vi "Generate Report work with Zee 2.vi"(6 "Graph Properties":T2(array[cluster])=[{"Plot Traces"=[{"Color Box"=4652800, "Boolean"=TRUE, "List 2"=39, "Boolean 2"=TRUE, "Boolean 3"=FALSE, "Offset"=0.0, "Gain"=1.0}, {"Color Box"=16733696, "Boolean"=TRUE, "List 2"=33, "Boolean 2"=FALSE, "Boolean 3"=FALSE, "Offset"=0.0, "Gain"=1.0}, {"Color Box"=393436, "Boolean"=TRUE, "List 2"=36, "Boolean 2"=FALSE, "Boolean 3"=FALSE, "Offset"=0.0, "Gain"=1.0}], "Gain Calculations"={"Threshold Trace"=39, "Min Thresh/%"=0.2, "Max Thresh/%"=0.8, "Gain calculated by dividing"=33, "Gain Range"=enum."Best Est", "Pre-peak-ms"=30.0, "by"=39}, "Impulse Plane"=enum."LARP", "Impulse Direction"=TRUE}, {"Plot Traces"=[{"Color Box"=4652800, "Boolean"=TRUE, "List 2"=39, "Boolean 2"=FALSE, "Boolean 3"=FALSE, "Offset"=0.0, "Gain"=1.0}, {"Color Box"=16733696, "Boolean"=TRUE, "List 2"=33, "Boolean 2"=TRUE, "Boolean 3"=FALSE, "Offset"=0.0, "Gain"=1.0}, {"Color Box"=393436, "Boolean"=TRUE, "List 2"=36, "Boolean 2"=TRUE, "Boolean 3"=FALSE, "Offset"=0.0, "Gain"=1.0}], "Gain Calculations"={"Threshold Trace"=39, "Min Thresh/%"=0.2, "Max Thresh/%"=0.8, "Gain calculated by dividing"=33, "Gain Range"=enum."Best Est", "Pre-peak-ms"=30.0, "by"=39}, "Impulse Plane"=enum."LARP", "Impulse Direction"=FALSE}, {"Plot Traces"=[{"Color Box"=4652800, "Boolean"=TRUE, "List 2"=42, "Boolean 2"=TRUE, "Boolean 3"=FALSE, "Offset"=0.0, "Gain"=1.0}, {"Color Box"=16733696, "Boolean"=TRUE, "List 2"=33, "Boolean 2"=FALSE, "Boolean 3"=FALSE, "Offset"=0.0, "Gain"=1.0}, {"Color Box"=393436, "Boolean"=TRUE, "List 2"=36, "Boolean 2"=FALSE, "Boolean 3"=FALSE, "Offset"=0.0, "Gain"=1.0}], "Gain Calculations"={"Threshold Trace"=42, "Min Thresh/%"=0.2, "Max Thresh/%"=0.8, "Gain calculated by dividing"=36, "Gain Range"=enum."Best Est", "Pre-peak-ms"=30.0, "by"=42}, "Impulse Plane"=enum."LARP", "Impulse Direction"=TRUE}, {"Plot Traces"=[{"Color Box"=4652800, "Boolean"=TRUE, "List 2"=42, "Boolean 2"=FALSE, "Boolean 3"=FALSE, "Offset"=0.0, "Gain"=1.0}, {"Color Box"=16733696, "Boolean"=TRUE, "List 2"=33, "Boolean 2"=TRUE, "Boolean 3"=FALSE, "Offset"=0.0, "Gain"=1.0}, {"Color Box"=393436, "Boolean"=TRUE, "List 2"=36, "Boolean 2"=TRUE, "Boolean 3"=FALSE, "Offset"=0.0, "Gain"=1.0}], "Gain Calculations"={"Threshold Trace"=42, "Min Thresh/%"=0.2, "Max Thresh/%"=0.8, "Gain calculated by dividing"=36, "Gain Range"=enum."Best Est", "Pre-peak-ms"=30.0, "by"=42}, "Impulse Plane"=enum."LARP", "Impulse Direction"=FALSE}, {"Plot Traces"=[{"Color Box"=4652800, "Boolean"=TRUE, "List 2"=38, "Boolean 2"=TRUE, "Boolean 3"=FALSE, "Offset"=0.0, "Gain"=1.0}, {"Color Box"=16733696, "Boolean"=TRUE, "List 2"=32, "Boolean 2"=FALSE, "Boolean 3"=FALSE, "Offset"=0.0, "Gain"=1.0}, {"Color Box"=393436, "Boolean"=TRUE, "List 2"=35, "Boolean 2"=FALSE, "Boolean 3"=FALSE, "Offset"=0.0, "Gain"=1.0}], "Gain Calculations"={"Threshold Trace"=38, "Min Thresh/%"=0.2, "Max Thresh/%"=0.8, "Gain calculated by dividing"=32, "Gain Range"=enum."Best Est", "Pre-peak-ms"=30.0, "by"=38}, "Impulse Plane"=enum."LARP", "Impulse Direction"=FALSE}, {"Plot Traces"=[{"Color Box"=4652800, "Boolean"=TRUE, "List 2"=38, "Boolean 2"=FALSE, "Boolean 3"=FALSE, "Offset"=0.0, "Gain"=1.0}, {"Color Box"=16733696, "Boolean"=TRUE, "List 2"=32, "Boolean 2"=TRUE, "Boolean 3"=FALSE, "Offset"=0.0, "Gain"=1.0}, {"Color Box"=393436, "Boolean"=TRUE, "List 2"=35, "Boolean 2"=TRUE, "Boolean 3"=FALSE, "Offset"=0.0, "Gain"=1.0}], "Gain Calculations"={"Threshold Trace"=38, "Min Thresh/%"=0.2, "Max Thresh/%"=0.8, "Gain calculated by dividing"=32, "Gain Range"=enum."Best Est", "Pre-peak-ms"=30.0, "by"=38}, "Impulse Plane"=enum."LARP", "Impulse Direction"=TRUE}, {"Plot Traces"=[{"Color Box"=4652800, "Boolean"=TRUE, "List 2"=41, "Boolean 2"=TRUE, "Boolean 3"=FALSE, "Offset"=0.0, "Gain"=1.0}, {"Color Box"=16733696, "Boolean"=TRUE, "List 2"=32, "Boolean 2"=FALSE, "Boolean 3"=FALSE, "Offset"=0.0, "Gain"=1.0}, {"Color Box"=393436, "Boolean"=TRUE, "List 2"=35, "Boolean 2"=FALSE, "Boolean 3"=FALSE, "Offset"=0.0, "Gain"=1.0}], "Gain Calculations"={"Threshold Trace"=41, "Min Thresh/%"=0.2, "Max Thresh/%"=0.8, "Gain calculated by dividing"=35, "Gain Range"=enum."Best Est", "Pre-peak-ms"=30.0, "by"=41}, "Impulse Plane"=enum."LARP", "Impulse Direction"=FALSE}, {"Plot Traces"=[{"Color Box"=4652800, "Boolean"=TRUE, "List 2"=41, "Boolean 2"=FALSE, "Boolean 3"=FALSE, "Offset"=0.0, "Gain"=1.0}, {"Color Box"=16733696, "Boolean"=TRUE, "List 2"=32, "Boolean 2"=TRUE, "Boolean 3"=FALSE, "Offset"=0.0, "Gain"=1.0}, {"Color Box"=393436, "Boolean"=TRUE, "List 2"=35, "Boolean 2"=TRUE, "Boolean 3"=FALSE, "Offset"=0.0, "Gain"=1.0}], "Gain Calculations"={"Threshold Trace"=41, "Min Thresh/%"=0.2, "Max Thresh/%"=0.8, "Gain calculated by dividing"=35, "Gain Range"=enum."Best Est", "Pre-peak-ms"=30.0, "by"=41}, "Impulse Plane"=enum."LARP", "Impulse Direction"=TRUE}, {"Plot Traces"=[{"Color Box"=4652800, "Boolean"=TRUE, "List 2"=39, "Boolean 2"=FALSE, "Boolean 3"=FALSE, "Offset"=0.0, "Gain"=1.0}, {"Color Box"=16733696, "Boolean"=TRUE, "List 2"=33, "Boolean 2"=TRUE, "Boolean 3"=FALSE, "Offset"=0.0, "Gain"=1.0}, {"Color Box"=393436, "Boolean"=TRUE, "List 2"=36, "Boolean 2"=TRUE, "Boolean 3"=FALSE, "Offset"=0.0, "Gain"=1.0}], "Gain Calculations"={"Threshold Trace"=39, "Min Thresh/%"=0.2, "Max Thresh/%"=0.8, "Gain calculated by dividing"=33, "Gain Range"=enum."Best Est", "Pre-peak-ms"=30.0, "by"=39}, "Impulse Plane"=enum."RALP", "Impulse Direction"=TRUE}, {"Plot Traces"=[{"Color Box"=4652800, "Boolean"=TRUE, "List 2"=39, "Boolean 2"=TRUE, "Boolean 3"=FALSE, "Offset"=0.0, "Gain"=1.0}, {"Color Box"=16733696, "Boolean"=TRUE, "List 2"=33, "Boolean 2"=FALSE, "Boolean 3"=FALSE, "Offset"=0.0, "Gain"=1.0}, {"Color Box"=393436, "Boolean"=TRUE, "List 2"=36, "Boolean 2"=FALSE, "Boolean 3"=FALSE, "Offset"=0.0, "Gain"=1.0}], "Gain Calculations"={"Threshold Trace"=39, "Min Thresh/%"=0.2, "Max Thresh/%"=0.8, "Gain calculated by dividing"=33, "Gain Range"=enum."Best Est", "Pre-peak-ms"=30.0, "by"=39}, "Impulse Plane"=enum."RALP", "Impulse Direction"=FALSE}, {"Plot Traces"=[{"Color Box"=4652800, "Boolean"=TRUE, "List 2"=42, "Boolean 2"=FALSE, "Boolean 3"=FALSE, "Offset"=0.0, "Gain"=1.0}, {"Color Box"=16733696, "Boolean"=TRUE, "List 2"=33, "Boolean 2"=TRUE, "Boolean 3"=FALSE, "Offset"=0.0, "Gain"=1.0}, {"Color Box"=393436, "Boolean"=TRUE, "List 2"=36, "Boolean 2"=TRUE, "Boolean 3"=FALSE, "Offset"=0.0, "Gain"=1.0}], "Gain Calculations"={"Threshold Trace"=42, "Min Thresh/%"=0.2, "Max Thresh/%"=0.8, "Gain calculated by dividing"=36, "Gain Range"=enum."Best Est", "Pre-peak-ms"=30.0, "by"=42}, "Impulse Plane"=enum."RALP", "Impulse Direction"=TRUE}, {"Plot Traces"=[{"Color Box"=4652800, "Boolean"=TRUE, "List 2"=42, "Boolean 2"=TRUE, "Boolean 3"=FALSE, "Offset"=0.0, "Gain"=1.0}, {"Color Box"=16733696, "Boolean"=TRUE, "List 2"=33, "Boolean 2"=FALSE, "Boolean 3"=FALSE, "Offset"=0.0, "Gain"=1.0}, {"Color Box"=393436, "Boolean"=TRUE, "List 2"=36, "Boolean 2"=FALSE, "Boolean 3"=FALSE, "Offset"=0.0, "Gain"=1.0}], "Gain Calculations"={"Threshold Trace"=42, "Min Thresh/%"=0.2, "Max Thresh/%"=0.8, "Gain calculated by dividing"=36, "Gain Range"=enum."Best Est", "Pre-peak-ms"=30.0, "by"=42}, "Impulse Plane"=enum."RALP", "Impulse Direction"=FALSE}, {"Plot Traces"=[{"Color Box"=4652800, "Boolean"=TRUE, "List 2"=38, "Boolean 2"=FALSE, "Boolean 3"=FALSE, "Offset"=0.0, "Gain"=1.0}, {"Color Box"=16733696, "Boolean"=TRUE, "List 2"=32, "Boolean 2"=TRUE, "Boolean 3"=FALSE, "Offset"=0.0, "Gain"=1.0}, {"Color Box"=393436, "Boolean"=TRUE, "List 2"=35, "Boolean 2"=TRUE, "Boolean 3"=FALSE, "Offset"=0.0, "Gain"=1.0}], "Gain Calculations"={"Threshold Trace"=38, "Min Thresh/%"=0.2, "Max Thresh/%"=0.8, "Gain calculated by dividing"=32, "Gain Range"=enum."Best Est", "Pre-peak-ms"=30.0, "by"=38}, "Impulse Plane"=enum."RALP", "Impulse Direction"=TRUE}, {"Plot Traces"=[{"Color Box"=4652800, "Boolean"=TRUE, "List 2"=38, "Boolean 2"=TRUE, "Boolean 3"=FALSE, "Offset"=0.0, "Gain"=1.0}, {"Color Box"=16733696, "Boolean"=TRUE, "List 2"=32, "Boolean 2"=FALSE, "Boolean 3"=FALSE, "Offset"=0.0, "Gain"=1.0}, {"Color Box"=393436, "Boolean"=TRUE, "List 2"=35, "Boolean 2"=FALSE, "Boolean 3"=FALSE, "Offset"=0.0, "Gain"=1.0}], "Gain Calculations"={"Threshold Trace"=38, "Min Thresh/%"=0.2, "Max Thresh/%"=0.8, "Gain calculated by dividing"=32, "Gain Range"=enum."Best Est", "Pre-peak-ms"=30.0, "by"=38}, "Impulse Plane"=enum."RALP", "Impulse Direction"=FALSE}, {"Plot Traces"=[{"Color Box"=4652800, "Boolean"=TRUE, "List 2"=41, "Boolean 2"=FALSE, "Boolean 3"=FALSE, "Offset"=0.0, "Gain"=1.0}, {"Color Box"=16733696, "Boolean"=TRUE, "List 2"=32, "Boolean 2"=TRUE, "Boolean 3"=FALSE, "Offset"=0.0, "Gain"=1.0}, {"Color Box"=393436, "Boolean"=TRUE, "List 2"=35, "Boolean 2"=TRUE, "Boolean 3"=FALSE, "Offset"=0.0, "Gain"=1.0}], "Gain Calculations"={"Threshold Trace"=41, "Min Thresh/%"=0.2, "Max Thresh/%"=0.8, "Gain calculated by dividing"=35, "Gain Range"=enum."Best Est", "Pre-peak-ms"=30.0, "by"=41}, "Impulse Plane"=enum."RALP", "Impulse Direction"=TRUE}, {"Plot Traces"=[{"Color Box"=4652800, "Boolean"=TRUE, "List 2"=41, "Boolean 2"=TRUE, "Boolean 3"=FALSE, "Offset"=0.0, "Gain"=1.0}, {"Color Box"=16733696, "Boolean"=TRUE, "List 2"=32, "Boolean 2"=FALSE, "Boolean 3"=FALSE, "Offset"=0.0, "Gain"=1.0}, {"Color Box"=393436, "Boolean"=TRUE, "List 2"=35, "Boolean 2"=FALSE, "Boolean 3"=FALSE, "Offset"=0.0, "Gain"=1.0}], "Gain Calculations"={"Threshold Trace"=41, "Min Thresh/%"=0.2, "Max Thresh/%"=0.8, "Gain calculated by dividing"=35, "Gain Range"=enum."Best Est", "Pre-peak-ms"=30.0, "by"=41}, "Impulse Plane"=enum."RALP", "Impulse Direction"=FALSE}] {"Gain Calculations"."by" items=["Hx Position-in-Head", "Hy Position-in-Head", "Hz Position-in-Head", "Hx Velocity-in-Head", "Hy Velocity-in-Head", "Hz Velocity-in-Head", "Hl Velocity-in-Head", "Hr Velocity-in-Head", "Lx Position-in-Head", "Ly Position-in-Head", "Lz Position-in-Head", "Lx Velocity-in-Head", "Ly Velocity-in-Head", "Lz Velocity-in-Head", "Ll Velocity-in-Head", "Lr Velocity-in-Head", "Rx Position-in-Head", "Ry Position-in-Head", "Rz Position-in-Head", "Rx Velocity-in-Head", "Ry Velocity-in-Head", "Rz Velocity-in-Head", "Rl Velocity-in-Head", "Rr Velocity-in-Head", "Button", "Ascension X", "Ascension X Vel", "Ascension Y", "Ascension Y Vel", "Ascension Z", "Ascension Z Vel", " ", "Lx Velocity-in-Eye", "Ly Velocity-in-Eye", "Lz Velocity-in-Eye", "Rx Velocity-in-Eye", "Ry Velocity-in-Eye", "Rz Velocity-in-Eye", "Hx Velocity-in-Left Eye", "Hy Velocity-in-Left Eye", "Hz Velocity-in-Left Eye", "Hx Velocity-in-Right-Eye", "Hy Velocity-in-Right-Eye", "Hz Velocity-in-Right-Eye"]; "Gain Calculations"."Pre-peak-ms" format="%.2f"; "Gain Calculations"."Gain calculated by dividing" items=["Hx Position-in-Head", "Hy Position-in-Head", "Hz Position-in-Head", "Hx Velocity-in-Head", "Hy Velocity-in-Head", "Hz Velocity-in-Head", "Hl Velocity-in-Head", "Hr Velocity-in-Head", "Lx Position-in-Head", "Ly Position-in-Head", "Lz Position-in-Head", "Lx Velocity-in-Head", "Ly Velocity-in-Head", "Lz Velocity-in-Head", "Ll Velocity-in-Head", "Lr Velocity-in-Head", "Rx Position-in-Head", "Ry Position-in-Head", "Rz Position-in-Head", "Rx Velocity-in-Head", "Ry Velocity-in-Head", "Rz Velocity-in-Head", "Rl Velocity-in-Head", "Rr Velocity-in-Head", "Button", "Ascension X", "Ascension X Vel", "Ascension Y", "Ascension Y Vel", "Ascension Z", "Ascension Z Vel", " ", "Lx Velocity-in-Eye", "Ly Velocity-in-Eye", "Lz Velocity-in-Eye", "Rx Velocity-in-Eye", "Ry Velocity-in-Eye", "Rz Velocity-in-Eye", "Hx Velocity-in-Left Eye", "Hy Velocity-in-Left Eye", "Hz Velocity-in-Left Eye", "Hx Velocity-in-Right-Eye", "Hy Velocity-in-Right-Eye", "Hz Velocity-in-Right-Eye"]; "Gain Calculations"."Max Thresh/%" format="%.2f"; "Gain Calculations"."Min Thresh/%" format="%.2f"; "Gain Calculations"."Threshold Trace" items=["Hx Position-in-Head", "Hy Position-in-Head", "Hz Position-in-Head", "Hx Velocity-in-Head", "Hy Velocity-in-Head", "Hz Velocity-in-Head", "Hl Velocity-in-Head", "Hr Velocity-in-Head", "Lx Position-in-Head", "Ly Position-in-Head", "Lz Position-in-Head", "Lx Velocity-in-Head", "Ly Velocity-in-Head", "Lz Velocity-in-Head", "Ll Velocity-in-Head", "Lr Velocity-in-Head", "Rx Position-in-Head", "Ry Position-in-Head", "Rz Position-in-Head", "Rx Velocity-in-Head", "Ry Velocity-in-Head", "Rz Velocity-in-Head", "Rl Velocity-in-Head", "Rr Velocity-in-Head", "Button", "Ascension X", "Ascension X Vel", "Ascension Y", "Ascension Y Vel", "Ascension Z", "Ascension Z Vel", " ", "Lx Velocity-in-Eye", "Ly Velocity-in-Eye", "Lz Velocity-in-Eye", "Rx Velocity-in-Eye", "Ry Velocity-in-Eye", "Rz Velocity-in-Eye", "Hx Velocity-in-Left Eye", "Hy Velocity-in-Left Eye", "Hz Velocity-in-Left Eye", "Hx Velocity-in-Right-Eye", "Hy Velocity-in-Right-Eye", "Hz Velocity-in-Right-Eye"]; "Plot Traces"."Gain" format="%.1f"; "Plot Traces"."Offset" format="%.1f"; "Plot Traces"."List 2" items=["Hx Position-in-Head", "Hy Position-in-Head", "Hz Position-in-Head", "Hx Velocity-in-Head", "Hy Velocity-in-Head", "Hz Velocity-in-Head", "Hl Velocity-in-Head", "Hr Velocity-in-Head", "Lx Position-in-Head", "Ly Position-in-Head", "Lz Position-in-Head", "Lx Velocity-in-Head", "Ly Velocity-in-Head", "Lz Velocity-in-Head", "Ll Velocity-in-Head", "Lr Velocity-in-Head", "Rx Position-in-Head", "Ry Position-in-Head", "Rz Position-in-Head", "Rx Velocity-in-Head", "Ry Velocity-in-Head", "Rz Velocity-in-Head", "Rl Velocity-in-Head", "Rr Velocity-in-Head", "Button", "Ascension X", "Ascension X Vel", "Ascension Y", "Ascension Y Vel", "Ascension Z", "Ascension Z Vel", " ", "Lx Velocity-in-Eye", "Ly Velocity-in-Eye", "Lz Velocity-in-Eye", "Rx Velocity-in-Eye", "Ry Velocity-in-Eye", "Rz Velocity-in-Eye", "Hx Velocity-in-Left Eye", "Hy Velocity-in-Left Eye", "Hz Velocity-in-Left Eye", "Hx Velocity-in-Right-Eye", "Hy Velocity-in-Right-Eye", "Hz Velocity-in-Right-Eye"]}, 8 "Impulse Positions":T4(array[cluster])=[{"Start"=5147, "End"=5187, "Impulse Plane"=enum."Yaw", "Impulse Direction +ve?"=TRUE, "Time offset"=0, "Amplitude offset"=0.0}, {"Start"=5544, "End"=5586, "Impulse Plane"=enum."Yaw", "Impulse Direction +ve?"=FALSE, "Time offset"=0, "Amplitude offset"=0.0}, {"Start"=5784, "End"=5826, "Impulse Plane"=enum."Yaw", "Impulse Direction +ve?"=FALSE, "Time offset"=0, "Amplitude offset"=0.0}, {"Start"=6210, "End"=6250, "Impulse Plane"=enum."Yaw", "Impulse Direction +ve?"=TRUE, "Time offset"=0, "Amplitude offset"=0.0}, {"Start"=6409, "End"=6449, "Impulse Plane"=enum."Yaw", "Impulse Direction +ve?"=TRUE, "Time offset"=0, "Amplitude offset"=0.0}, {"Start"=6617, "End"=6657, "Impulse Plane"=enum."Yaw", "Impulse Direction +ve?"=TRUE, "Time offset"=0, "Amplitude offset"=0.0}, {"Start"=6856, "End"=6898, "Impulse Plane"=enum."Yaw", "Impulse Direction +ve?"=FALSE, "Time offset"=0, "Amplitude offset"=0.0}, {"Start"=7143, "End"=7185, "Impulse Plane"=enum."Yaw", "Impulse Direction +ve?"=FALSE, "Time offset"=0, "Amplitude offset"=0.0}, {"Start"=7918, "End"=7958, "Impulse Plane"=enum."Yaw", "Impulse Direction +ve?"=TRUE, "Time offset"=0, "Amplitude offset"=0.0}, {"Start"=8170, "End"=8210, "Impulse Plane"=enum."Yaw", "Impulse Direction +ve?"=TRUE, "Time offset"=0, "Amplitude offset"=0.0}, {"Start"=9145, "End"=9185, "Impulse Plane"=enum."Yaw", "Impulse Direction +ve?"=TRUE, "Time offset"=0, "Amplitude offset"=0.0}, {"Start"=9434, "End"=9476, "Impulse Plane"=enum."Yaw", "Impulse Direction +ve?"=FALSE, "Time offset"=0, "Amplitude offset"=0.0}, {"Start"=9732, "End"=9774, "Impulse Plane"=enum."Yaw", "Impulse Direction +ve?"=FALSE, "Time offset"=0, "Amplitude offset"=0.0}, {"Start"=10023, "End"=10065, "Impulse Plane"=enum."Yaw", "Impulse Direction +ve?"=FALSE, "Time offset"=0, "Amplitude offset"=0.0}, {"Start"=10545, "End"=10585, "Impulse Plane"=enum."Yaw", "Impulse Direction +ve?"=TRUE, "Time offset"=0, "Amplitude offset"=0.0}, {"Start"=11028, "End"=11068, "Impulse Plane"=enum."Yaw", "Impulse Direction +ve?"=TRUE, "Time offset"=0, "Amplitude offset"=0.0}, {"Start"=11326, "End"=11366, "Impulse Plane"=enum."Yaw", "Impulse Direction +ve?"=TRUE, "Time offset"=0, "Amplitude offset"=0.0}, {"Start"=11654, "End"=11696, "Impulse Plane"=enum."Yaw", "Impulse Direction +ve?"=FALSE, "Time offset"=0, "Amplitude offset"=0.0}, {"Start"=11983, "End"=12025, "Impulse Plane"=enum."Yaw", "Impulse Direction +ve?"=FALSE, "Time offset"=0, "Amplitude offset"=0.0}, {"Start"=12228, "End"=12270, "Impulse Plane"=enum."Yaw", "Impulse Direction +ve?"=FALSE, "Time offset"=0, "Amplitude offset"=0.0}, {"Start"=12796, "End"=12836, "Impulse Plane"=enum."Yaw", "Impulse Direction +ve?"=TRUE, "Time offset"=0, "Amplitude offset"=0.0}, {"Start"=13150, "End"=13190, "Impulse Plane"=enum."Yaw", "Impulse Direction +ve?"=TRUE, "Time offset"=0, "Amplitude offset"=0.0}, {"Start"=13420, "End"=13460, "Impulse Plane"=enum."Yaw", "Impulse Direction +ve?"=TRUE, "Time offset"=0, "Amplitude offset"=0.0}, {"Start"=14002, "End"=14044, "Impulse Plane"=enum."Yaw", "Impulse Direction +ve?"=FALSE, "Time offset"=0, "Amplitude offset"=0.0}, {"Start"=14311, "End"=14351, "Impulse Plane"=enum."Yaw", "Impulse Direction +ve?"=TRUE, "Time offset"=0, "Amplitude offset"=0.0}, {"Start"=14611, "End"=14651, "Impulse Plane"=enum."Yaw", "Impulse Direction +ve?"=TRUE, "Time offset"=0, "Amplitude offset"=0.0}, {"Start"=15419, "End"=15461, "Impulse Plane"=enum."Yaw", "Impulse Direction +ve?"=FALSE, "Time offset"=0, "Amplitude offset"=0.0}, {"Start"=15681, "End"=15723, "Impulse Plane"=enum."Yaw", "Impulse Direction +ve?"=FALSE, "Time offset"=0, "Amplitude offset"=0.0}, {"Start"=15969, "End"=16009, "Impulse Plane"=enum."Yaw", "Impulse Direction +ve?"=TRUE, "Time offset"=0, "Amplitude offset"=0.0}, {"Start"=16818, "End"=16858, "Impulse Plane"=enum."Yaw", "Impulse Direction +ve?"=TRUE, "Time offset"=0, "Amplitude offset"=0.0}, {"Start"=17055, "End"=17097, "Impulse Plane"=enum."Yaw", "Impulse Direction +ve?"=FALSE, "Time offset"=0, "Amplitude offset"=0.0}, {"Start"=18327, "End"=18369, "Impulse Plane"=enum."Yaw", "Impulse Direction +ve?"=FALSE, "Time offset"=0, "Amplitude offset"=0.0}, {"Start"=18817, "End"=18859, "Impulse Plane"=enum."Yaw", "Impulse Direction +ve?"=FALSE, "Time offset"=0, "Amplitude offset"=0.0}, {"Start"=19049, "End"=19089, "Impulse Plane"=enum."Yaw", "Impulse Direction +ve?"=TRUE, "Time offset"=0, "Amplitude offset"=0.0}, {"Start"=21122, "End"=21188, "Impulse Plane"=enum."LARP", "Impulse Direction +ve?"=TRUE, "Time offset"=0, "Amplitude offset"=0.0}, {"Start"=21362, "End"=21430, "Impulse Plane"=enum."LARP", "Impulse Direction +ve?"=TRUE, "Time offset"=0, "Amplitude offset"=0.0}, {"Start"=21593, "End"=21661, "Impulse Plane"=enum."LARP", "Impulse Direction +ve?"=TRUE, "Time offset"=0, "Amplitude offset"=0.0}, {"Start"=22327, "End"=22395, "Impulse Plane"=enum."LARP", "Impulse Direction +ve?"=TRUE, "Time offset"=0, "Amplitude offset"=0.0}, {"Start"=22537, "End"=22604, "Impulse Plane"=enum."LARP", "Impulse Direction +ve?"=TRUE, "Time offset"=0, "Amplitude offset"=0.0}, {"Start"=22777, "End"=22844, "Impulse Plane"=enum."LARP", "Impulse Direction +ve?"=TRUE, "Time offset"=0, "Amplitude offset"=0.0}, {"Start"=23019, "End"=23086, "Impulse Plane"=enum."LARP", "Impulse Direction +ve?"=TRUE, "Time offset"=0, "Amplitude offset"=0.0}, {"Start"=23291, "End"=23358, "Impulse Plane"=enum."LARP", "Impulse Direction +ve?"=TRUE, "Time offset"=0, "Amplitude offset"=0.0}, {"Start"=23566, "End"=23631, "Impulse Plane"=enum."LARP", "Impulse Direction +ve?"=TRUE, "Time offset"=0, "Amplitude offset"=0.0}, {"Start"=23861, "End"=23929, "Impulse Plane"=enum."LARP", "Impulse Direction +ve?"=FALSE, "Time offset"=0, "Amplitude offset"=0.0}, {"Start"=24575, "End"=24641, "Impulse Plane"=enum."LARP", "Impulse Direction +ve?"=TRUE, "Time offset"=0, "Amplitude offset"=0.0}, {"Start"=24924, "End"=24993, "Impulse Plane"=enum."LARP", "Impulse Direction +ve?"=TRUE, "Time offset"=0, "Amplitude offset"=0.0}, {"Start"=25253, "End"=25318, "Impulse Plane"=enum."LARP", "Impulse Direction +ve?"=TRUE, "Time offset"=0, "Amplitude offset"=0.0}, {"Start"=25536, "End"=25602, "Impulse Plane"=enum."LARP", "Impulse Direction +ve?"=TRUE, "Time offset"=0, "Amplitude offset"=0.0}, {"Start"=26288, "End"=26350, "Impulse Plane"=enum."LARP", "Impulse Direction +ve?"=FALSE, "Time offset"=0, "Amplitude offset"=0.0}, {"Start"=26578, "End"=26645, "Impulse Plane"=enum."LARP", "Impulse Direction +ve?"=FALSE, "Time offset"=0, "Amplitude offset"=0.0}, {"Start"=26940, "End"=27006, "Impulse Plane"=enum."LARP", "Impulse Direction +ve?"=FALSE, "Time offset"=0, "Amplitude offset"=0.0}, {"Start"=27202, "End"=27271, "Impulse Plane"=enum."LARP", "Impulse Direction +ve?"=FALSE, "Time offset"=0, "Amplitude offset"=0.0}, {"Start"=27477, "End"=27544, "Impulse Plane"=enum."LARP", "Impulse Direction +ve?"=TRUE, "Time offset"=0, "Amplitude offset"=0.0}, {"Start"=27709, "End"=27775, "Impulse Plane"=enum."LARP", "Impulse Direction +ve?"=TRUE, "Time offset"=0, "Amplitude offset"=0.0}, {"Start"=27926, "End"=27993, "Impulse Plane"=enum."LARP", "Impulse Direction +ve?"=TRUE, "Time offset"=0, "Amplitude offset"=0.0}, {"Start"=28185, "End"=28251, "Impulse Plane"=enum."LARP", "Impulse Direction +ve?"=TRUE, "Time offset"=0, "Amplitude offset"=0.0}, {"Start"=28672, "End"=28736, "Impulse Plane"=enum."LARP", "Impulse Direction +ve?"=FALSE, "Time offset"=0, "Amplitude offset"=0.0}, {"Start"=29607, "End"=29677, "Impulse Plane"=enum."LARP", "Impulse Direction +ve?"=TRUE, "Time offset"=0, "Amplitude offset"=0.0}, {"Start"=29829, "End"=29898, "Impulse Plane"=enum."LARP", "Impulse Direction +ve?"=TRUE, "Time offset"=0, "Amplitude offset"=0.0}, {"Start"=30266, "End"=30335, "Impulse Plane"=enum."LARP", "Impulse Direction +ve?"=TRUE, "Time offset"=0, "Amplitude offset"=0.0}, {"Start"=30991, "End"=31057, "Impulse Plane"=enum."LARP", "Impulse Direction +ve?"=FALSE, "Time offset"=0, "Amplitude offset"=0.0}, {"Start"=32437, "End"=32505, "Impulse Plane"=enum."LARP", "Impulse Direction +ve?"=TRUE, "Time offset"=0, "Amplitude offset"=0.0}, {"Start"=33030, "End"=33097, "Impulse Plane"=enum."LARP", "Impulse Direction +ve?"=FALSE, "Time offset"=0, "Amplitude offset"=0.0}, {"Start"=33660, "End"=33727, "Impulse Plane"=enum."LARP", "Impulse Direction +ve?"=FALSE, "Time offset"=0, "Amplitude offset"=0.0}, {"Start"=34390, "End"=34456, "Impulse Plane"=enum."LARP", "Impulse Direction +ve?"=FALSE, "Time offset"=0, "Amplitude offset"=0.0}, {"Start"=34672, "End"=34738, "Impulse Plane"=enum."LARP", "Impulse Direction +ve?"=FALSE, "Time offset"=0, "Amplitude offset"=0.0}, {"Start"=34936, "End"=35002, "Impulse Plane"=enum."LARP", "Impulse Direction +ve?"=FALSE, "Time offset"=0, "Amplitude offset"=0.0}, {"Start"=35914, "End"=35980, "Impulse Plane"=enum."LARP", "Impulse Direction +ve?"=TRUE, "Time offset"=0, "Amplitude offset"=0.0}, {"Start"=39368, "End"=39431, "Impulse Plane"=enum."RALP", "Impulse Direction +ve?"=TRUE, "Time offset"=0, "Amplitude offset"=0.0}, {"Start"=39786, "End"=39846, "Impulse Plane"=enum."RALP", "Impulse Direction +ve?"=FALSE, "Time offset"=0, "Amplitude offset"=0.0}, {"Start"=40447, "End"=40509, "Impulse Plane"=enum."RALP", "Impulse Direction +ve?"=FALSE, "Time offset"=0, "Amplitude offset"=0.0}, {"Start"=41117, "End"=41187, "Impulse Plane"=enum."RALP", "Impulse Direction +ve?"=TRUE, "Time offset"=0, "Amplitude offset"=0.0}, {"Start"=41617, "End"=41683, "Impulse Plane"=enum."RALP", "Impulse Direction +ve?"=TRUE, "Time offset"=0, "Amplitude offset"=0.0}, {"Start"=41887, "End"=41955, "Impulse Plane"=enum."RALP", "Impulse Direction +ve?"=TRUE, "Time offset"=0, "Amplitude offset"=0.0}, {"Start"=43772, "End"=43831, "Impulse Plane"=enum."RALP", "Impulse Direction +ve?"=FALSE, "Time offset"=0, "Amplitude offset"=0.0}, {"Start"=44057, "End"=44115, "Impulse Plane"=enum."RALP", "Impulse Direction +ve?"=FALSE, "Time offset"=0, "Amplitude offset"=0.0}, {"Start"=44373, "End"=44430, "Impulse Plane"=enum."RALP", "Impulse Direction +ve?"=FALSE, "Time offset"=0, "Amplitude offset"=0.0}, {"Start"=45082, "End"=45151, "Impulse Plane"=enum."RALP", "Impulse Direction +ve?"=TRUE, "Time offset"=0, "Amplitude offset"=0.0}, {"Start"=45381, "End"=45447, "Impulse Plane"=enum."RALP", "Impulse Direction +ve?"=TRUE, "Time offset"=0, "Amplitude offset"=0.0}, {"Start"=45691, "End"=45755, "Impulse Plane"=enum."RALP", "Impulse Direction +ve?"=TRUE, "Time offset"=0, "Amplitude offset"=0.0}, {"Start"=46038, "End"=46104, "Impulse Plane"=enum."RALP", "Impulse Direction +ve?"=TRUE, "Time offset"=0, "Amplitude offset"=0.0}, {"Start"=46642, "End"=46702, "Impulse Plane"=enum."RALP", "Impulse Direction +ve?"=FALSE, "Time offset"=0, "Amplitude offset"=0.0}, {"Start"=46873, "End"=46933, "Impulse Plane"=enum."RALP", "Impulse Direction +ve?"=FALSE, "Time offset"=0, "Amplitude offset"=0.0}, {"Start"=47122, "End"=47182, "Impulse Plane"=enum."RALP", "Impulse Direction +ve?"=FALSE, "Time offset"=0, "Amplitude offset"=0.0}, {"Start"=47662, "End"=47727, "Impulse Plane"=enum."RALP", "Impulse Direction +ve?"=TRUE, "Time offset"=0, "Amplitude offset"=0.0}, {"Start"=47923, "End"=47990, "Impulse Plane"=enum."RALP", "Impulse Direction +ve?"=TRUE, "Time offset"=0, "Amplitude offset"=0.0}, {"Start"=48188, "End"=48255, "Impulse Plane"=enum."RALP", "Impulse Direction +ve?"=TRUE, "Time offset"=0, "Amplitude offset"=0.0}, {"Start"=48495, "End"=48562, "Impulse Plane"=enum."RALP", "Impulse Direction +ve?"=TRUE, "Time offset"=0, "Amplitude offset"=0.0}, {"Start"=48819, "End"=48877, "Impulse Plane"=enum."RALP", "Impulse Direction +ve?"=FALSE, "Time offset"=0, "Amplitude offset"=0.0}, {"Start"=49036, "End"=49095, "Impulse Plane"=enum."RALP", "Impulse Direction +ve?"=FALSE, "Time offset"=0, "Amplitude offset"=0.0}, {"Start"=49258, "End"=49318, "Impulse Plane"=enum."RALP", "Impulse Direction +ve?"=FALSE, "Time offset"=0, "Amplitude offset"=0.0}, {"Start"=49479, "End"=49537, "Impulse Plane"=enum."RALP", "Impulse Direction +ve?"=FALSE, "Time offset"=0, "Amplitude offset"=0.0}, {"Start"=49905, "End"=49969, "Impulse Plane"=enum."RALP", "Impulse Direction +ve?"=TRUE, "Time offset"=0, "Amplitude offset"=0.0}, {"Start"=50154, "End"=50219, "Impulse Plane"=enum."RALP", "Impulse Direction +ve?"=TRUE, "Time offset"=0, "Amplitude offset"=0.0}, {"Start"=50398, "End"=50461, "Impulse Plane"=enum."RALP", "Impulse Direction +ve?"=TRUE, "Time offset"=0, "Amplitude offset"=0.0}, {"Start"=50655, "End"=50719, "Impulse Plane"=enum."RALP", "Impulse Direction +ve?"=TRUE, "Time offset"=0, "Amplitude offset"=0.0}, {"Start"=50933, "End"=51000, "Impulse Plane"=enum."RALP", "Impulse Direction +ve?"=TRUE, "Time offset"=0, "Amplitude offset"=0.0}, {"Start"=51274, "End"=51333, "Impulse Plane"=enum."RALP", "Impulse Direction +ve?"=FALSE, "Time offset"=0, "Amplitude offset"=0.0}, {"Start"=51504, "End"=51564, "Impulse Plane"=enum."RALP", "Impulse Direction +ve?"=FALSE, "Time offset"=0, "Amplitude offset"=0.0}, {"Start"=52162, "End"=52224, "Impulse Plane"=enum."RALP", "Impulse Direction +ve?"=FALSE, "Time offset"=0, "Amplitude offset"=0.0}, {"Start"=52733, "End"=52798, "Impulse Plane"=enum."RALP", "Impulse Direction +ve?"=TRUE, "Time offset"=0, "Amplitude offset"=0.0}, {"Start"=52999, "End"=53070, "Impulse Plane"=enum."RALP", "Impulse Direction +ve?"=TRUE, "Time offset"=0, "Amplitude offset"=0.0}, {"Start"=53554, "End"=53614, "Impulse Plane"=enum."RALP", "Impulse Direction +ve?"=FALSE, "Time offset"=0, "Amplitude offset"=0.0}, {"Start"=54009, "End"=54075, "Impulse Plane"=enum."RALP", "Impulse Direction +ve?"=TRUE, "Time offset"=0, "Amplitude offset"=0.0}, {"Start"=54306, "End"=54369, "Impulse Plane"=enum."RALP", "Impulse Direction +ve?"=TRUE, "Time offset"=0, "Amplitude offset"=0.0}, {"Start"=57322, "End"=57372, "Impulse Plane"=enum."Pitch", "Impulse Direction +ve?"=TRUE, "Time offset"=0, "Amplitude offset"=0.0}, {"Start"=57651, "End"=57714, "Impulse Plane"=enum."Pitch", "Impulse Direction +ve?"=FALSE, "Time offset"=0, "Amplitude offset"=0.0}, {"Start"=59751, "End"=59813, "Impulse Plane"=enum."Pitch", "Impulse Direction +ve?"=FALSE, "Time offset"=0, "Amplitude offset"=0.0}, {"Start"=60061, "End"=60111, "Impulse Plane"=enum."Pitch", "Impulse Direction +ve?"=TRUE, "Time offset"=0, "Amplitude offset"=0.0}, {"Start"=60325, "End"=60375, "Impulse Plane"=enum."Pitch", "Impulse Direction +ve?"=TRUE, "Time offset"=0, "Amplitude offset"=0.0}, {"Start"=60782, "End"=60832, "Impulse Plane"=enum."Pitch", "Impulse Direction +ve?"=TRUE, "Time offset"=0, "Amplitude offset"=0.0}, {"Start"=61083, "End"=61133, "Impulse Plane"=enum."Pitch", "Impulse Direction +ve?"=TRUE, "Time offset"=0, "Amplitude offset"=0.0}, {"Start"=61454, "End"=61517, "Impulse Plane"=enum."RALP", "Impulse Direction +ve?"=FALSE, "Time offset"=0, "Amplitude offset"=0.0}, {"Start"=61774, "End"=61839, "Impulse Plane"=enum."Pitch", "Impulse Direction +ve?"=FALSE, "Time offset"=0, "Amplitude offset"=0.0}, {"Start"=62617, "End"=62681, "Impulse Plane"=enum."Pitch", "Impulse Direction +ve?"=FALSE, "Time offset"=0, "Amplitude offset"=0.0}, {"Start"=62970, "End"=63029, "Impulse Plane"=enum."RALP", "Impulse Direction +ve?"=FALSE, "Time offset"=0, "Amplitude offset"=0.0}, {"Start"=63322, "End"=63372, "Impulse Plane"=enum."Pitch", "Impulse Direction +ve?"=TRUE, "Time offset"=0, "Amplitude offset"=0.0}, {"Start"=63812, "End"=63874, "Impulse Plane"=enum."Pitch", "Impulse Direction +ve?"=FALSE, "Time offset"=0, "Amplitude offset"=0.0}, {"Start"=64056, "End"=64106, "Impulse Plane"=enum."Pitch", "Impulse Direction +ve?"=TRUE, "Time offset"=0, "Amplitude offset"=0.0}, {"Start"=64345, "End"=64395, "Impulse Plane"=enum."Pitch", "Impulse Direction +ve?"=TRUE, "Time offset"=0, "Amplitude offset"=0.0}, {"Start"=64579, "End"=64642, "Impulse Plane"=enum."Pitch", "Impulse Direction +ve?"=FALSE, "Time offset"=0, "Amplitude offset"=0.0}, {"Start"=65064, "End"=65124, "Impulse Plane"=enum."Pitch", "Impulse Direction +ve?"=FALSE, "Time offset"=0, "Amplitude offset"=0.0}, {"Start"=65293, "End"=65343, "Impulse Plane"=enum."Pitch", "Impulse Direction +ve?"=TRUE, "Time offset"=0, "Amplitude offset"=0.0}, {"Start"=65517, "End"=65567, "Impulse Plane"=enum."Pitch", "Impulse Direction +ve?"=TRUE, "Time offset"=0, "Amplitude offset"=0.0}, {"Start"=65777, "End"=65840, "Impulse Plane"=enum."Pitch", "Impulse Direction +ve?"=FALSE, "Time offset"=0, "Amplitude offset"=0.0}, {"Start"=66097, "End"=66147, "Impulse Plane"=enum."Pitch", "Impulse Direction +ve?"=TRUE, "Time offset"=0, "Amplitude offset"=0.0}, {"Start"=66404, "End"=66466, "Impulse Plane"=enum."Pitch", "Impulse Direction +ve?"=FALSE, "Time offset"=0, "Amplitude offset"=0.0}, {"Start"=66652, "End"=66702, "Impulse Plane"=enum."Pitch", "Impulse Direction +ve?"=TRUE, "Time offset"=0, "Amplitude offset"=0.0}, {"Start"=66952, "End"=67015, "Impulse Plane"=enum."Pitch", "Impulse Direction +ve?"=FALSE, "Time offset"=0, "Amplitude offset"=0.0}, {"Start"=67449, "End"=67499, "Impulse Plane"=enum."Pitch", "Impulse Direction +ve?"=TRUE, "Time offset"=0, "Amplitude offset"=0.0}, {"Start"=67699, "End"=67749, "Impulse Plane"=enum."Pitch", "Impulse Direction +ve?"=TRUE, "Time offset"=0, "Amplitude offset"=0.0}, {"Start"=67929, "End"=67994, "Impulse Plane"=enum."Pitch", "Impulse Direction +ve?"=FALSE, "Time offset"=0, "Amplitude offset"=0.0}, {"Start"=68411, "End"=68461, "Impulse Plane"=enum."Pitch", "Impulse Direction +ve?"=TRUE, "Time offset"=0, "Amplitude offset"=0.0}, {"Start"=68634, "End"=68684, "Impulse Plane"=enum."Pitch", "Impulse Direction +ve?"=TRUE, "Time offset"=0, "Amplitude offset"=0.0}, {"Start"=68900, "End"=68959, "Impulse Plane"=enum."RALP", "Impulse Direction +ve?"=FALSE, "Time offset"=0, "Amplitude offset"=0.0}, {"Start"=69109, "End"=69159, "Impulse Plane"=enum."Pitch", "Impulse Direction +ve?"=TRUE, "Time offset"=0, "Amplitude offset"=0.0}, {"Start"=69322, "End"=69384, "Impulse Plane"=enum."Pitch", "Impulse Direction +ve?"=FALSE, "Time offset"=0, "Amplitude offset"=0.0}, {"Start"=69544, "End"=69594, "Impulse Plane"=enum."Pitch", "Impulse Direction +ve?"=TRUE, "Time offset"=0, "Amplitude offset"=0.0}, {"Start"=69759, "End"=69809, "Impulse Plane"=enum."Pitch", "Impulse Direction +ve?"=TRUE, "Time offset"=0, "Amplitude offset"=0.0}, {"Start"=70027, "End"=70090, "Impulse Plane"=enum."Pitch", "Impulse Direction +ve?"=FALSE, "Time offset"=0, "Amplitude offset"=0.0}, {"Start"=70267, "End"=70334, "Impulse Plane"=enum."RALP", "Impulse Direction +ve?"=TRUE, "Time offset"=0, "Amplitude offset"=0.0}, {"Start"=70534, "End"=70595, "Impulse Plane"=enum."Pitch", "Impulse Direction +ve?"=FALSE, "Time offset"=0, "Amplitude offset"=0.0}, {"Start"=76740, "End"=76805, "Impulse Plane"=enum."Roll", "Impulse Direction +ve?"=TRUE, "Time offset"=0, "Amplitude offset"=0.0}, {"Start"=77174, "End"=77234, "Impulse Plane"=enum."Roll", "Impulse Direction +ve?"=TRUE, "Time offset"=0, "Amplitude offset"=0.0}, {"Start"=77525, "End"=77586, "Impulse Plane"=enum."Roll", "Impulse Direction +ve?"=FALSE, "Time offset"=0, "Amplitude offset"=0.0}, {"Start"=79364, "End"=79424, "Impulse Plane"=enum."Roll", "Impulse Direction +ve?"=TRUE, "Time offset"=0, "Amplitude offset"=0.0}, {"Start"=80141, "End"=80199, "Impulse Plane"=enum."Roll", "Impulse Direction +ve?"=FALSE, "Time offset"=0, "Amplitude offset"=0.0}, {"Start"=80380, "End"=80441, "Impulse Plane"=enum."Roll", "Impulse Direction +ve?"=FALSE, "Time offset"=0, "Amplitude offset"=0.0}, {"Start"=81556, "End"=81616, "Impulse Plane"=enum."Roll", "Impulse Direction +ve?"=TRUE, "Time offset"=0, "Amplitude offset"=0.0}, {"Start"=81786, "End"=81847, "Impulse Plane"=enum."Roll", "Impulse Direction +ve?"=TRUE, "Time offset"=0, "Amplitude offset"=0.0}, {"Start"=83326, "End"=83386, "Impulse Plane"=enum."Roll", "Impulse Direction +ve?"=TRUE, "Time offset"=0, "Amplitude offset"=0.0}, {"Start"=86069, "End"=86127, "Impulse Plane"=enum."Roll", "Impulse Direction +ve?"=TRUE, "Time offset"=0, "Amplitude offset"=0.0}, {"Start"=87195, "End"=87253, "Impulse Plane"=enum."RALP", "Impulse Direction +ve?"=FALSE, "Time offset"=0, "Amplitude offset"=0.0}, {"Start"=87769, "End"=87831, "Impulse Plane"=enum."Roll", "Impulse Direction +ve?"=TRUE, "Time offset"=0, "Amplitude offset"=0.0}, {"Start"=88236, "End"=88293, "Impulse Plane"=enum."Roll", "Impulse Direction +ve?"=TRUE, "Time offset"=0, "Amplitude offset"=0.0}, {"Start"=88481, "End"=88542, "Impulse Plane"=enum."Roll", "Impulse Direction +ve?"=TRUE, "Time offset"=0, "Amplitude offset"=0.0}, {"Start"=90160, "End"=90222, "Impulse Plane"=enum."Roll", "Impulse Direction +ve?"=TRUE, "Time offset"=0, "Amplitude offset"=0.0}] {"Amplitude offset" format="%.2f"}, 9 "Impulse Data":T3 {"Data Channels" format="%.2f"}) -> ()   [LabVIEW 2013, in "generate report.lvlib"]
uses:
  generate report.lvlib
  comm/impulse/impulse functions.lvlib
panel:
  in  "Means":bool
  in  "Target Position":T1(ring)
  in  "Subject ID":enum16{"dsz", "nbs", "jpc", "aam", "mcs", "rac"}(ring)
  in  "Save to File":bool
  in  "stop":bool
  # "Copyright Americo A. Migliaccio (c) 2002 All Rights Reserved by Author"
  # "-"
  # "+"
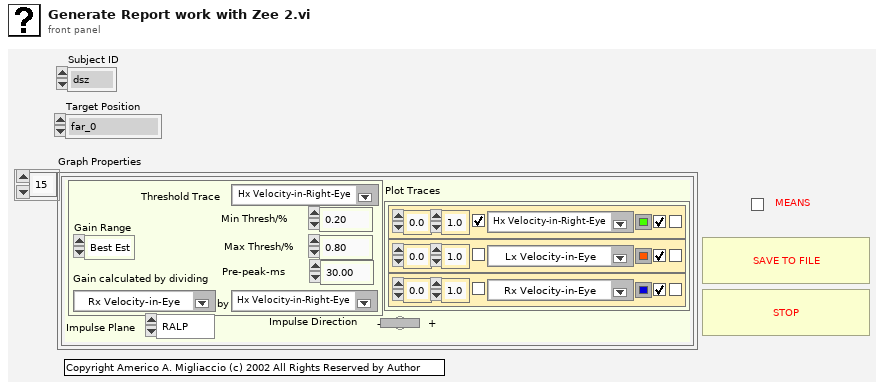
[diagram p1: front panel]
types:
  T1 = enum16{"far_0", "far_left_20", "far_left_30", "far_right_20", "far_right_30", "near_0", "near_left_20", "near_right_20"}
  T2 = cluster{"Plot Traces":cluster{"Color Box":u32, "Boolean":bool, "List 2":u16, "Boolean 2":bool, "Boolean 3":bool, "Offset":dbl, "Gain":dbl}[], "Gain Calculations":cluster{"Threshold Trace":u16, "Min Thresh/%":dbl, "Max Thresh/%":dbl, "Gain calculated by dividing":u16, "Gain Range":enum16{"Peak %", "Best Est", "Thresh"}, "Pre-peak-ms":dbl, "by":u16}, "Impulse Plane":enum16{"Other", "Yaw", "Pitch", "Roll", "LARP", "RALP"}, "Impulse Direction":bool}[]
  T3 = cluster{"Data Channels":dbl[][], "Sample Rate":i32, "Channel List":string[]}
  T4 = cluster{"Start":i32, "End":i32, "Impulse Plane":enum16{"Other", "Yaw", "Pitch", "Roll", "LARP", "RALP"}, "Impulse Direction +ve?":bool, "Time offset":i32, "Amplitude offset":dbl}[]
  T5 = enum16{"open", "open or create", "create or replace", "create", "open (read only)"}
  T6 = enum16{"Other", "Yaw", "Pitch", "Roll", "LARP", "RALP"}
  T7 = cluster{"Color Box":u32, "Boolean":bool, "List 2":u16, "Boolean 2":bool, "Boolean 3":bool, "Offset":dbl, "Gain":dbl}[]
  T8 = cluster{"Threshold Trace":u16, "Min Thresh/%":dbl, "Max Thresh/%":dbl, "Gain calculated by dividing":u16, "Gain Range":enum16{"Peak %", "Best Est", "Thresh"}, "Pre-peak-ms":dbl, "by":u16}
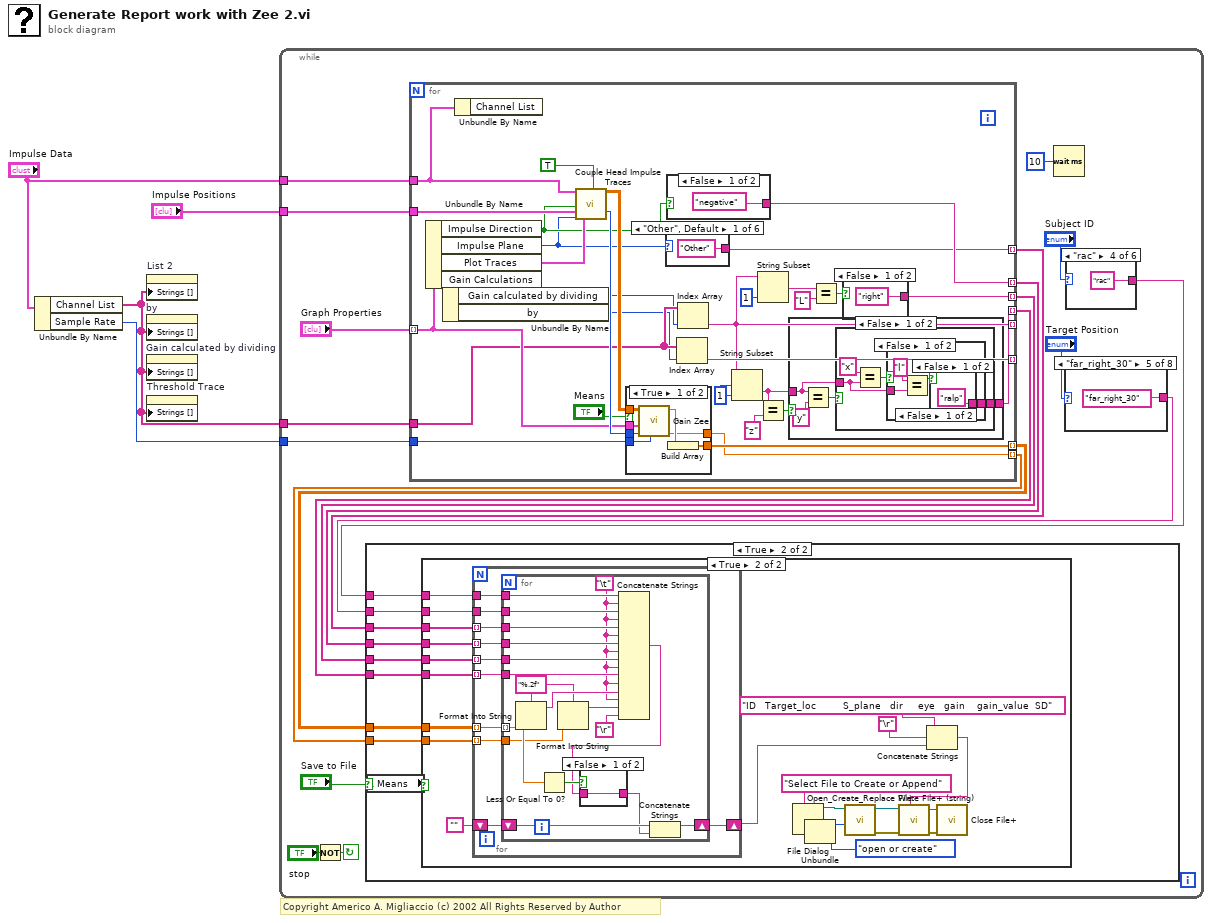
[diagram p0: block diagram]
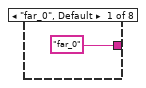
[diagram p2: hidden frame]
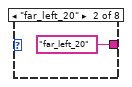
[diagram p3: hidden frame]
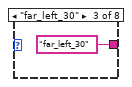
[diagram p4: hidden frame]
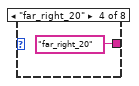
[diagram p5: hidden frame]
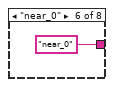
[diagram p6: hidden frame]
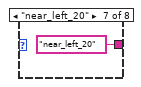
[diagram p7: hidden frame]
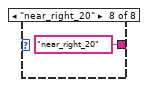
[diagram p8: hidden frame]
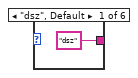
[diagram p9: hidden frame]
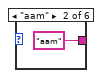
[diagram p10: hidden frame]
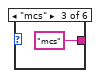
[diagram p11: hidden frame]
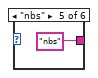
[diagram p12: hidden frame]
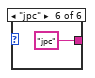
[diagram p13: hidden frame]
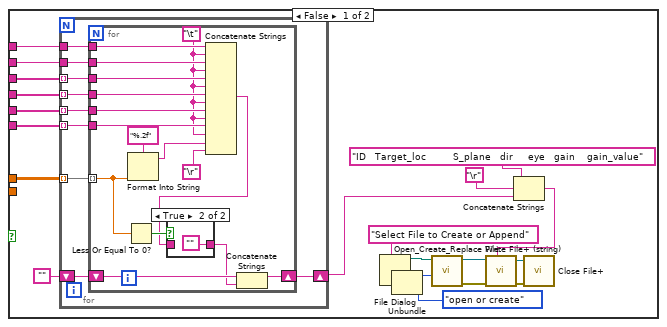
[diagram p15: hidden frame]
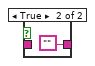
[diagram p17: hidden frame]
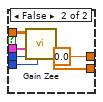
[diagram p18: hidden frame]
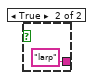
[diagram p19: hidden frame]
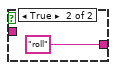
[diagram p20: hidden frame]
diagram:
  # "Copyright Americo A. Migliaccio (c) 2002 All Rights Reserved by Author"
  n1 = Unbundle By Name("Impulse Data") -> ("Channel List"=w1:string[], "Sample Rate"=w3:i32)
  n2 = property on="List 2" class="Ring (strict)"("Strings []"=w1) -> ()  [unwired: 2 in, 2 out]
  n3 = property on="by" class="Ring (strict)"("Strings []"=w1) -> ()  [unwired: 2 in, 2 out]
  n4 = property on="Gain calculated by dividing" class="Ring (strict)"("Strings []"=w1) -> ()  [unwired: 2 in, 2 out]
  n5 = property on="Threshold Trace" class="Ring (strict)"("Strings []"=w1) -> ()  [unwired: 2 in, 2 out]
  n6 = while {
    tunnel: w3 -> [w21]
    tunnel: "Impulse Positions" -> [w22]
    tunnel: "Impulse Data" -> [w23]
    tunnel: w1 -> [w17]
    stop <- w18 continue-if-true
    n7 = Not(x="stop") -> (.not. x?=w18:bool)
    n8 = for {
      tunnel: "Graph Properties" -> [w171] mode=indexing
      tunnel: w22 -> [w175]
      tunnel: w23 -> [w168]
      tunnel: w21 -> [w170]
      tunnel: [w158] -> w16 mode=indexing
      tunnel: w17 -> [w166]
      tunnel: [w153] -> _ mode=indexing
      tunnel: [w163] -> _ mode=indexing
      tunnel: [w161] -> w13 mode=indexing
      tunnel: [w160] -> w12 mode=indexing
      tunnel: [w154] -> w7 mode=indexing
      tunnel: [w147] -> w6 mode=indexing
      tunnel: [w146] -> w5 mode=indexing
      w152 = 1 ("length (rest)")
      n9 = Unbundle By Name(w171) -> ("Impulse Direction"=w162:bool, "Impulse Plane"=w159:T6, "Plot Traces"=w172:T7, "Gain Calculations"=w167:T8)
      n10 = Unbundle By Name(w167) -> ("Gain calculated by dividing"=w165:u16, "by"=w164:u16)
      n11 = Unbundle By Name(w168) -> ()  [unwired: 1 out]
      n12 = call "Couple Head Impulse Traces.vi"("Data Input"=w168, "Impulse Positions"=w175, "Impulse Direction +ve?"=w162, "Impulse Plane"=w159, "Plot Selection 2"=w172, "Interpolate"=TRUE) -> ("No Impulses"=w173:i32, "Impulses"=w174:dbl[][])  [unwired: 10 in, 2 out]
      n13 = case shown="True" "Means" {
        tunnel: w174 -> [w182 w188]
        tunnel: w173 -> [w181 w187]
        tunnel: w171 -> [w180 w186]
        tunnel: w170 -> [w179 w185]
        tunnel: [w177 w184] -> w160
        tunnel: [w176 0.0 ("STD")] -> w146
        frame True {
          n14 = call "Gain Zee.vi"("Sample Rate"=w179, "Number of Impulses"=w181, "Graph Cluster"=w180, "Data (in)"=w182) -> ("STD"=w176:dbl, "GAIN"=w178:dbl)  [unwired: 3 in, 1 out]
          n15 = Build Array(w178) -> (w177:dbl[])
        }
        frame False {
          n16 = call "Gain Zee.vi"("Sample Rate"=w185, "Number of Impulses"=w187, "Graph Cluster"=w186, "Data (in)"=w188) -> ("STD array"=w184:dbl[])  [unwired: 3 in, 2 out]
        }
      }
      n17 = case shown="\"Other\", Default" w159 {
        tunnel: ["Other" "yaw" "pitch" "roll" "larp" "ralp"] -> w158
        frame "Other", Default {
        }
        frame "Yaw" {
        }
        frame "Pitch" {
        }
        frame "Roll" {
        }
        frame "LARP" {
        }
        frame "RALP" {
        }
      }
      n18 = case shown="False" w162 {
        tunnel: ["negative" "positive"] -> w161
        frame False {
        }
        frame True {
        }
      }
      n19 = Index Array(array=w166, index=w164) -> (element=w163:string)
      n20 = Index Array(array=w166, index=w165) -> (element=w153:string)
      n21 = String Subset(string=w153, offset (0)=w152, length (rest)=w152) -> (substring=w148:string)
      n22 = String Subset(string=w153, length (rest)=1 ("length (rest)")) -> (substring=w156:string)  [unwired: 1 in]
      n23 = Equal?(x=w148, y="z") -> (x = y?=w150:bool)
      n24 = case shown="False" w150 {
        tunnel: [w190 "hor"] -> w147
        tunnel: w148 -> [w189 _]
        frame False {
          n25 = Equal?(x=w189, y="y") -> (x = y?=w191:bool)
          n26 = case shown="False" w191 {
            tunnel: [w194 "pitch"] -> w190
            tunnel: w189 -> [w193 _]
            frame False {
              n27 = Equal?(x="x" ("y"), y=w193) -> (x = y?=w195:bool)
              n28 = case shown="False" w195 {
                tunnel: [w198 "roll"] -> w194
                tunnel: w193 -> [w200 _]
                frame False {
                  n29 = Equal?(x="l" ("y"), y=w200) -> (x = y?=w197:bool)
                  n30 = case shown="False" w197 {
                    tunnel: ["ralp" ("y") "larp" ("y")] -> w198
                    frame False {
                    }
                    frame True {
                    }
                  }
                }
                frame True {
                }
              }
            }
            frame True {
            }
          }
        }
        frame True {
        }
      }
      n31 = Equal?(x=w156, y="L") -> (x = y?=w151:bool)
      n32 = case shown="False" w151 {
        tunnel: ["right" "left"] -> w154
        frame False {
        }
        frame True {
        }
      }
    }
    n33 = Wait (ms)(milliseconds to wait=u32 10) -> ()  [unwired: 1 out]
    n34 = case shown="\"far_right_30\"" "Target Position" {
      tunnel: ["far_0" "far_left_20" "far_left_30" "far_right_20" "far_right_30" "near_0" "near_left_20" "near_right_20"] -> w9
      frame "far_0", Default {
      }
      frame "far_left_20" {
      }
      frame "far_left_30" {
      }
      frame "far_right_20" {
      }
      frame "far_right_30" {
      }
      frame "near_0" {
      }
      frame "near_left_20" {
      }
      frame "near_right_20" {
      }
    }
    n35 = case shown="\"rac\"" "Subject ID" {
      tunnel: ["dsz" "aam" "mcs" "rac" "nbs" "jpc"] -> w8
      frame "dsz", Default {
      }
      frame "aam" {
      }
      frame "mcs" {
      }
      frame "rac" {
      }
      frame "nbs" {
      }
      frame "jpc" {
      }
    }
    n36 = case shown="True" "Save to File" {
      tunnel: w16 -> [_ w46]
      tunnel: w13 -> [_ w45]
      tunnel: w12 -> [_ w44]
      tunnel: w9 -> [_ w42]
      tunnel: w8 -> [_ w43]
      tunnel: w7 -> [_ w41]
      tunnel: w6 -> [_ w40]
      tunnel: w5 -> [_ w39]
      frame False {
      }
      frame True {
        n37 = local read "Means"() -> (w38:bool)
        n38 = case shown="True" w38 {
          tunnel: w46 -> [w66 w114]
          tunnel: w45 -> [w53 w101]
          tunnel: w44 -> [w52 w100]
          tunnel: w43 -> [w51 w99]
          tunnel: w42 -> [w50 w98]
          tunnel: w41 -> [w49 w97]
          tunnel: w40 -> [w48 w96]
          tunnel: w39 -> [_ w95]
          frame False {
            n39 = for {
              tunnel: w66 -> [w75] mode=indexing
              shift-right: [w72] -> w54
              shift-left: "" -> [w73]
              tunnel: w53 -> [w74] mode=indexing
              tunnel: w52 -> [w71] mode=indexing
              tunnel: w51 -> [w70]
              tunnel: w50 -> [w69]
              tunnel: w49 -> [w68] mode=indexing
              tunnel: w48 -> [w67] mode=indexing
              n40 = for {
                tunnel: w75 -> [w82]
                tunnel: w74 -> [w83]
                shift-right: [w90] -> w72
                shift-left: w73 -> [w87]
                tunnel: w71 -> [w89] mode=indexing
                tunnel: w70 -> [w85]
                tunnel: w69 -> [w84]
                tunnel: w68 -> [w81]
                tunnel: w67 -> [w80]
                w79 = "\t"
                n41 = Less Or Equal To 0?(x=w89) -> (x <= 0?=w88:bool)
                n42 = Format Into String(format string="%.2f", w89) -> (resulting string=w76:string)  [unwired: 2 in, 1 out]
                n43 = Concatenate Strings(w85, w79, w84, w79, w82, w79, w83, w79, w81, w79, w80, w79, w76, "\r") -> (w78:string)
                n44 = case shown="True" w88 {
                  tunnel: w78 -> [w92 _]
                  tunnel: [w92 ""] -> w86
                  frame False {
                  }
                  frame True {
                  }
                }
                n45 = Concatenate Strings(w87, w86) -> (w90:string)
              }
            }
            n46 = File Dialog(7:"Select File to Create or Append" ("prompt")) -> (0:w47:errorcluster, 3:w62:path)  [unwired: 6 in, 2 out]
            n47 = Unbundle(w47) -> ()  [unwired: 3 out]
            n48 = call <vilib>:"Open_Create_Replace File.vi"("function (open:0)"=T5."open or create", "file path"=w62) -> ("error out"=w64:errorcluster, "refnum"=w63:refnum<file>)  [unwired: 6 in, 2 out]
            n49 = Concatenate Strings("ID   Target_loc         S_plane   dir     eye   gain    gain_value" ("prompt"), "\r", w54) -> (w58:string)
            n50 = call <vilib>:"Write File+ (string).vi"("string"=w58, "error in (no error)"=w64, "refnum"=w63) -> ("error out"=w60:errorcluster, "dup refnum"=w61:refnum<file>)  [unwired: 4 in, 1 out]
            n51 = call <vilib>:"Close File+.vi"("error in (no error)"=w60, "refnum"=w61) -> ()  [unwired: 3 in, 3 out]
          }
          frame True {
            n52 = for {
              tunnel: w114 -> [w124] mode=indexing
              shift-right: [w121] -> w102
              shift-left: "" -> [w122]
              tunnel: w101 -> [w123] mode=indexing
              tunnel: w100 -> [w120] mode=indexing
              tunnel: w99 -> [w119]
              tunnel: w98 -> [w118]
              tunnel: w97 -> [w117] mode=indexing
              tunnel: w96 -> [w116] mode=indexing
              tunnel: w95 -> [w115] mode=indexing
              n53 = for {
                tunnel: w124 -> [w134]
                tunnel: w123 -> [w135]
                shift-right: [w142] -> w121
                shift-left: w122 -> [w139]
                tunnel: w120 -> [w141] mode=indexing
                tunnel: w119 -> [w137]
                tunnel: w118 -> [w136]
                tunnel: w117 -> [w133]
                tunnel: w116 -> [w132]
                tunnel: w115 -> [w125]
                w129 = "\t"
                w127 = "%.2f" ("format string")
                n54 = Format Into String(format string=w127, w141) -> (resulting string=w130:string)  [unwired: 2 in, 1 out]
                n55 = Less Or Equal To 0?(x=w141) -> (x <= 0?=w140:bool)
                n56 = Format Into String(format string=w127, w125) -> (resulting string=w126:string)  [unwired: 2 in, 1 out]
                n57 = Concatenate Strings(w137, w129, w136, w129, w134, w129, w135, w129, w133, w129, w132, w129, w130, w129, w126, "\r") -> (w131:string)
                n58 = case shown="False" w140 {
                  tunnel: w131 -> [w143 _]
                  tunnel: [w143 ""] -> w138
                  frame False {
                  }
                  frame True {
                  }
                }
                n59 = Concatenate Strings(w139, w138) -> (w142:string)
              }
            }
            n60 = File Dialog(7:"Select File to Create or Append" ("prompt")) -> (0:w94:errorcluster, 3:w110:path)  [unwired: 6 in, 2 out]
            n61 = Unbundle(w94) -> ()  [unwired: 3 out]
            n62 = call <vilib>:"Open_Create_Replace File.vi"("function (open:0)"=T5."open or create", "file path"=w110) -> ("error out"=w112:errorcluster, "refnum"=w111:refnum<file>)  [unwired: 6 in, 2 out]
            n63 = Concatenate Strings("ID   Target_loc         S_plane   dir     eye   gain    gain_value  SD" ("prompt"), "\r", w102) -> (w106:string)
            n64 = call <vilib>:"Write File+ (string).vi"("string"=w106, "error in (no error)"=w112, "refnum"=w111) -> ("error out"=w108:errorcluster, "dup refnum"=w109:refnum<file>)  [unwired: 4 in, 1 out]
            n65 = call <vilib>:"Close File+.vi"("error in (no error)"=w108, "refnum"=w109) -> ()  [unwired: 3 in, 3 out]
          }
        }
      }
    }
  }
